vi "MW contrast over time.vi"() -> ()   [LabVIEW 2012]
panel:
  in  "stop":bool
  out "Waveform Graph":dbl[](graph)
  in  "Time":dbl
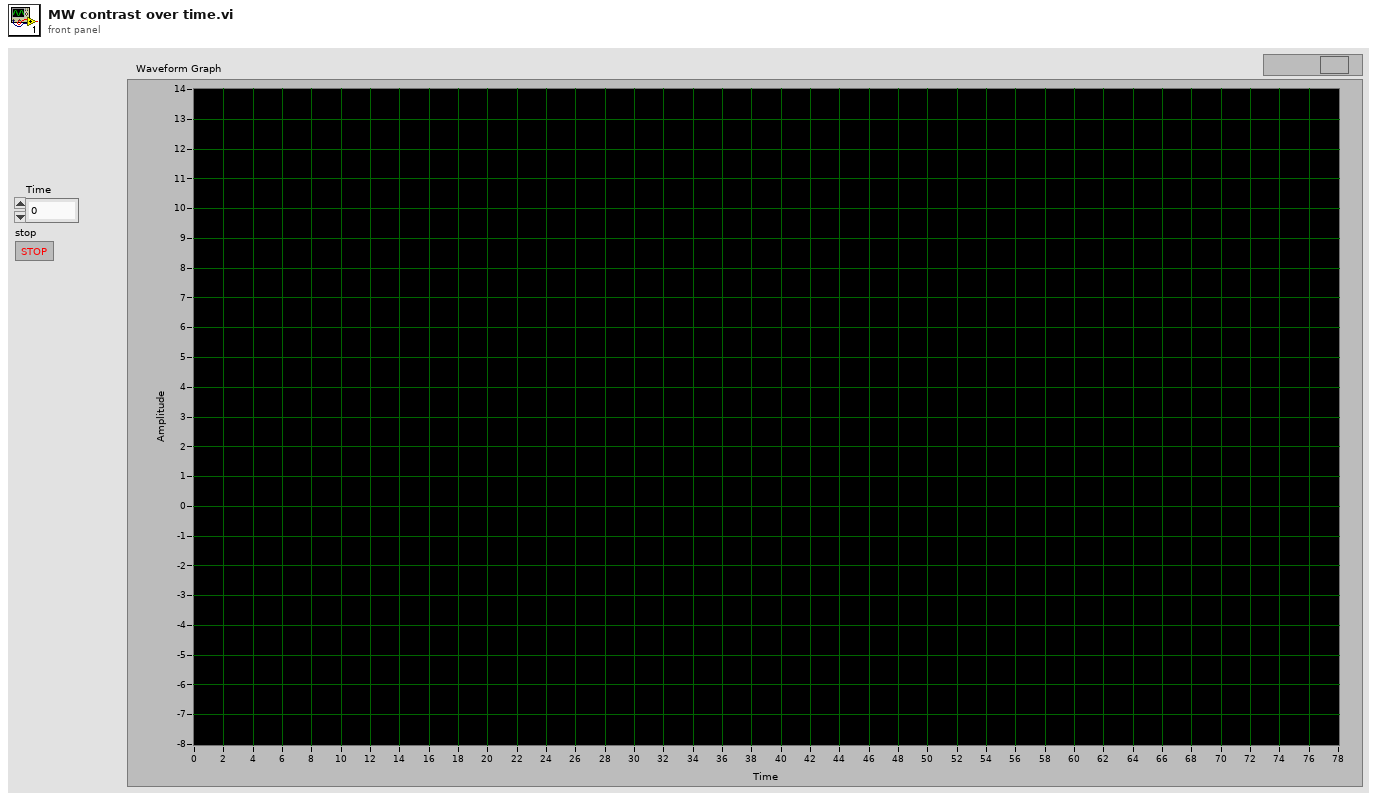
[diagram p1: front panel]
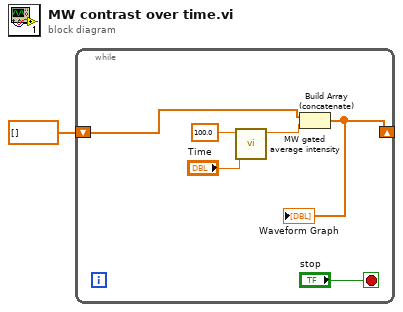
[diagram p0: block diagram]
diagram:
  n1 = while {
    shift-right: [w3] -> _
    shift-left: dbl[] [] -> [w4]
    stop <- "stop" stop-if-true
    n2 = call "MW gated average intensity.vi"("Time"="Time", "rate"=100.0) -> ("Contrast (%)"=w5:dbl)  [unwired: 9 in]
    n3 = Build Array (concatenate)(w4, w5) -> (w3:dbl[])
    "Waveform Graph" <- w3
  }
